vi "main_symulacyjny.vi"() -> ()   [LabVIEW 2020]
uses:
  Kontrolki/Parametry_cosinusow.ctl
  Kontrolki/Parametry_cosinusa.ctl
  Kontrolki/Rodzaj_wzmacniacza.ctl
  Kontrolki/Rodzaj_modulacji.ctl
  Kontrolki/Dane.ctl
  Kontrolki/Pasmo_przenoszenia.ctl
  <vilib>/measure/maspectr.llb/FFT Spectrum (Mag-Phase) for 1 Chan.vi
  <vilib>/measure/NI_MAPro.lvlib
panel:
  out "Widmo_sygnalu_zdemodulowanego":cluster{"f0":dbl, "df":dbl, "magnitude":dbl[]}(graph)
  out "Moc_szczytowa":dbl
  out "Sprawnosc":dbl
  out "Moc_srednia":dbl
  out "Energia_sygnalu_zmodulowanego":waveform(dbl)(graph) caption="Waveform Chart 2"
  out "Moc_sygnalu_zmodulowanego":waveform(dbl)(graph) caption="Waveform Chart 2"
  out "Widmo_sygnalu_zmodulowanego":cluster{"f0":dbl, "df":dbl, "magnitude":dbl[]}(graph)
  out "Sygnal_zmodulowany":waveform(dbl)(graph) caption="Waveform Chart 2"
  out "Widmo_sygnalu_modulujacego":cluster{"f0":dbl, "df":dbl, "magnitude":dbl[]}(graph)
  out "Sygnal_modulujacy_i_zdemodulowany":waveform(dbl)[](graph) caption="Waveform Chart 2"
  in  "Rodzaj_modulacji":T1
  in  "Parametry_sygnalu_nosnego":T2={"Amplituda [V]"=1.0, "Czestotliwosc [Hz] "=2.0, "Faza [rad]"=0.0}
  in  "Rodzaj_wzmacniacza":T3
  in  "Wzmocnienie":dbl=1.0
  in  "Milisekund_na_dane":u32=20
  in  "Parametry_sygnalu_modulujacego":T4 {"Czestotliwosc [Hz]" min=0.3 step=0.1}
  in  "stop":bool
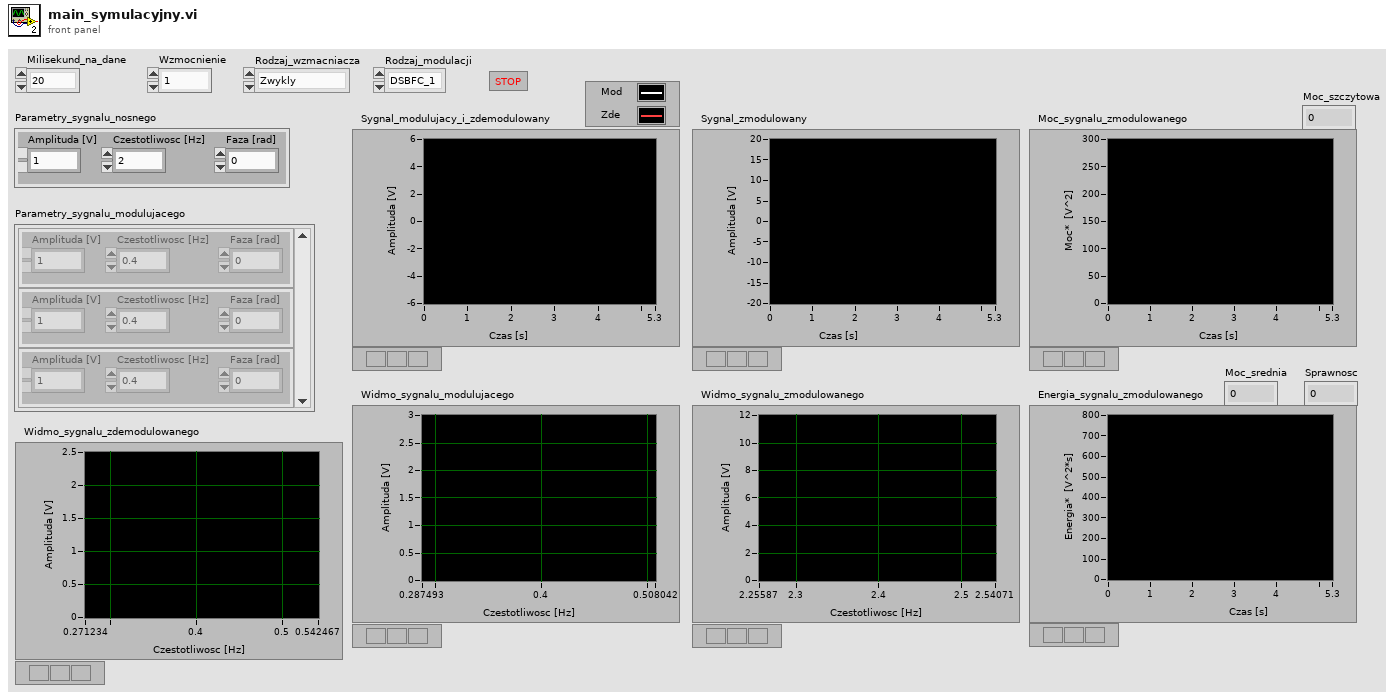
[diagram p1: front panel]
types:
  T1 = typedef "Rodzaj_modulacji.ctl" = enum16{"DSBFC_1", "DSBFC_2", "DSBSC", "USSBSC", "LSSBSC"}
  T2 = typedef "Parametry_cosinusa.ctl" = cluster{"Amplituda [V]":dbl, "Czestotliwosc [Hz] ":dbl, "Faza [rad]":dbl}
  T3 = typedef "Rodzaj_wzmacniacza.ctl" = enum16{"Zwykly", "Calkujacy", "Rozniczkujacy"}
  T4 = typedef "Parametry_cosinusow.ctl" = T2[]
  T5 = typedef "Dane.ctl" = cluster{"Parametry_sygnalu_modulujacego":T4, "Parametry_sygnalu_modulujacego_przesunietego":T4, "Sygnal_modulujacy_wzmocniony":dbl[], "Milisekund_na_dane":u32, "Wzmocnienie":dbl, "Rodzaj_wzmacniacza":T3, "Parametry_sygnalu_nosnego":T2, "Wektor_czasu":dbl[], "Sygnal_zmodulowany":dbl[], "Moc_sygnalu":dbl[], "Energia_sygnalu":dbl[], "Moc_szczytowa":dbl, "Sprawnosc":dbl, "Wartosc_poprzednia":dbl, "Czas":dbl, "Rodzaj_modulacji":T1, "Wartosc_poprzednia 2":dbl, "Moc_srednia":dbl, "Sygnal_zdemodulowany":dbl[], "Pasmo_przenoszenia":T6, "Rzeczywisty_sygnal":dbl[], "Rzeczywisty_zmodulowany":dbl[]}
  T6 = typedef "Pasmo_przenoszenia.ctl" = cluster{"f_L":dbl, "f_H":dbl}
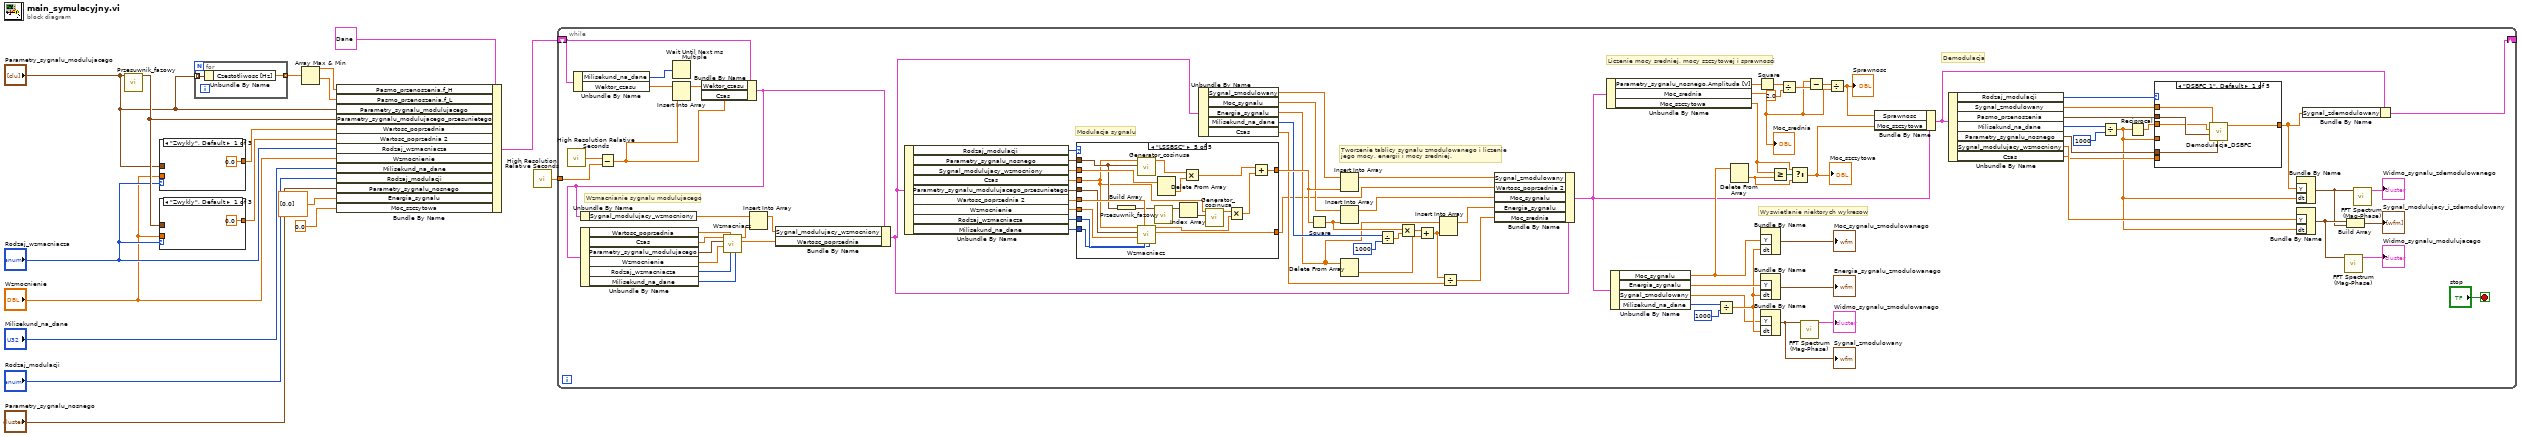
[diagram p0: block diagram]
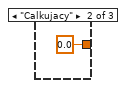
[diagram p2: hidden frame]
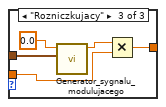
[diagram p3: hidden frame]
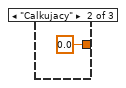
[diagram p4: hidden frame]
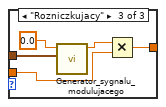
[diagram p5: hidden frame]
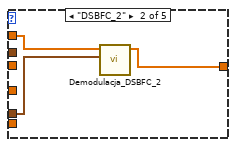
[diagram p6: hidden frame]
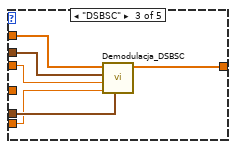
[diagram p7: hidden frame]
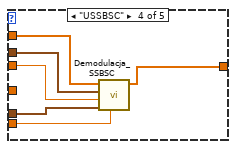
[diagram p8: hidden frame]
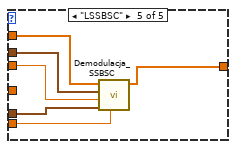
[diagram p9: hidden frame]
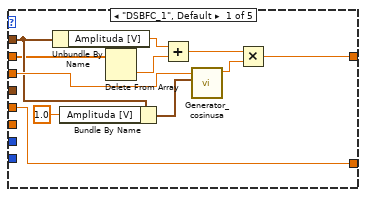
[diagram p10: hidden frame]
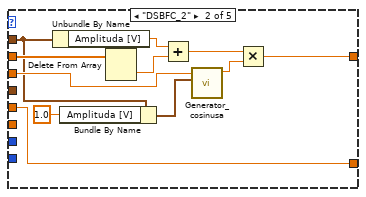
[diagram p11: hidden frame]
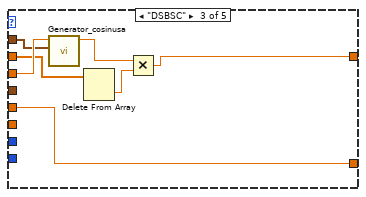
[diagram p12: hidden frame]
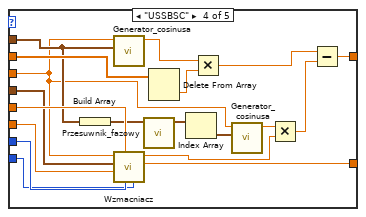
[diagram p13: hidden frame]
diagram:
  n1 = call "Przesuwnik_fazowy.vi"("Parametry_cosinusow"="Parametry_sygnalu_modulujacego") -> ("Parametry_cosinusow\nprzesuniete_w_fazie"=w9:T2[])  [unwired: 10 in]
  n2 = case shown="\"Zwykly\", Default" "Rodzaj_wzmacniacza" {
    tunnel: "Parametry_sygnalu_modulujacego" -> [_ _ w24]
    tunnel: [0.0 ("Sygnal_modulujacy") 0.0 ("Sygnal_modulujacy") w21] -> w11
    tunnel: "Wzmocnienie" -> [_ _ w20]
    frame "Zwykly", Default {
    }
    frame "Calkujacy" {
    }
    frame "Rozniczkujacy" {
      n3 = call "Generator_sygnalu_modulujacego.vi"("Parametry_cosinusow"=w24, "Czas"=0.0) -> ("Sygnal_modulujacy"=w22:dbl)  [unwired: 9 in]
      n4 = Multiply(x=w22, y=w20) -> (x*y=w21:dbl)
    }
  }
  n5 = case shown="\"Zwykly\", Default" "Rodzaj_wzmacniacza" {
    tunnel: w9 -> [_ _ w31]
    tunnel: [0.0 ("Sygnal_modulujacy") 0.0 ("Sygnal_modulujacy") w29] -> w10
    tunnel: "Wzmocnienie" -> [_ _ w27]
    frame "Zwykly", Default {
    }
    frame "Calkujacy" {
    }
    frame "Rozniczkujacy" {
      n6 = call "Generator_sygnalu_modulujacego.vi"("Parametry_cosinusow"=w31, "Czas"=0.0) -> ("Sygnal_modulujacy"=w28:dbl)  [unwired: 9 in]
      n7 = Multiply(x=w28, y=w27) -> (x*y=w29:dbl)
    }
  }
  n8 = for {
    tunnel: "Parametry_sygnalu_modulujacego" -> [w33] mode=indexing
    tunnel: [w32] -> w3 mode=indexing
    n9 = Unbundle By Name(w33) -> ("Czestotliwosc [Hz]"=w32:dbl)
  }
  n10 = Array Max & Min(array=w3) -> (max value=w1:dbl, min value=w2:dbl)  [unwired: 2 out]
  n11 = Bundle By Name(cluster=T5 {"Parametry_sygnalu_modulujacego"=[], "Parametry_sygnalu_modulujacego_przesunietego"=[], "Sygnal_modulujacy_wzmocniony"=[], "Milisekund_na_dane"=0, "Wzmocnienie"=0.0, "Rodzaj_wzmacniacza"=enum."Zwykly", "Parametry_sygnalu_nosnego"={"Amplituda [V]"=0.0, "Czestotliwosc [Hz] "=0.0, "Faza [rad]"=0.0}, "Wektor_czasu"=[], "Sygnal_zmodulowany"=[], "Moc_sygnalu"=[], "Energia_sygnalu"=[], "Moc_szczytowa"=0.0, "Sprawnosc"=0.0, "Wartosc_poprzednia"=0.0, "Czas"=0.0, "Rodzaj_modulacji"=enum."DSBFC_1", "Wartosc_poprzednia 2"=0.0, "Moc_srednia"=0.0, "Sygnal_zdemodulowany"=[], "Pasmo_przenoszenia"={"f_L"=0.0, "f_H"=0.0}, "Rzeczywisty_sygnal"=[], "Rzeczywisty_zmodulowany"=[]} ("Dane"), "Pasmo_przenoszenia.f_H"=w1, "Pasmo_przenoszenia.f_L"=w2, "Parametry_sygnalu_modulujacego"="Parametry_sygnalu_modulujacego", "Parametry_sygnalu_modulujacego_przesunietego"=w9, "Wartosc_poprzednia"=w11, "Wartosc_poprzednia 2"=w10, "Rodzaj_wzmacniacza"="Rodzaj_wzmacniacza", "Wzmocnienie"="Wzmocnienie", "Milisekund_na_dane"="Milisekund_na_dane", "Rodzaj_modulacji"="Rodzaj_modulacji", "Parametry_sygnalu_nosnego"="Parametry_sygnalu_nosnego", "Energia_sygnalu"=dbl[] [0.0], "Moc_szczytowa"=0.0) -> (w14:T5)
  n12 = call <vilib>:"High Resolution Relative Seconds.vi"() -> ("relative seconds"=w13:dbl)
  n13 = while {
    shift-right: [w37] -> _
    shift-left: w14 -> [w114]
    tunnel: w13 -> [w118]
    stop <- "stop" stop-if-true
    # "Wzmacnianie sygnalu modulujacego"
    # "Liczenie mocy sredniej, mocy szczytowej i sprawnosci"
    # "Wyswietlanie niektorych wykresow"
    # "Tworzenie tablicy sygnalu zmodulowanego i liczenie\njego mocy, energii i mocy sredniej."
    # "Demodulacja"
    # "Modulacja sygnalu"
    n14 = call <vilib>:"High Resolution Relative Seconds.vi"() -> ("relative seconds"=w119:dbl)
    n15 = Unbundle By Name(w114) -> ("Milisekund_na_dane"=w115:u32, "Wektor_czasu"=w117:dbl[])
    n16 = Subtract(x=w119, y=w118) -> (x-y=w113:dbl)
    n17 = Wait Until Next ms Multiple(millisecond multiple=w115) -> ()  [unwired: 1 out]
    n18 = Insert Into Array(array=w117, new element=w113) -> (w116:dbl[])  [unwired: 1 in]
    n19 = Bundle By Name(cluster=w114, "Wektor_czasu"=w116, "Czas"=w113) -> (w100:T5)
    n20 = Unbundle By Name(w100) -> ("Wartosc_poprzednia"=w112:dbl, "Czas"=w93:dbl, "Parametry_sygnalu_modulujacego"=w92:T4, "Wzmocnienie"=w109:dbl, "Rodzaj_wzmacniacza"=w110:T3, "Milisekund_na_dane"=w111:u32)
    n21 = Unbundle By Name(w100) -> ("Sygnal_modulujacy_wzmocniony"=w99:dbl[])
    n22 = call "Wzmacniacz.vi"("Milisekund_na_dane"=w111, "Rodzaj_wzmacniacza"=w110, "Wartosc_poprzednia"=w112, "Wzmocnienie"=w109, "Parametry_cosinusow"=w92, "Czas"=w93) -> ("Wartosc_poprzednia"=w91:dbl, "Sygnal_wzmocniony"=w90:dbl)  [unwired: 4 in]
    n23 = Insert Into Array(array=w99, new element=w90) -> (w98:dbl[])  [unwired: 1 in]
    n24 = Bundle By Name(cluster=w100, "Sygnal_modulujacy_wzmocniony"=w98, "Wartosc_poprzednia"=w91) -> (w97:T5)
    n25 = Unbundle By Name(w97) -> ("Rodzaj_modulacji"=w105:T1, "Parametry_sygnalu_nosnego"=w108:T2, "Sygnal_modulujacy_wzmocniony"=w96:dbl[], "Czas"=w107:dbl, "Parametry_sygnalu_modulujacego_przesunietego"=w106:T4, "Wartosc_poprzednia 2"=w104:dbl, "Wzmocnienie"=w103:dbl, "Rodzaj_wzmacniacza"=w102:T3, "Milisekund_na_dane"=w101:u32)
    n26 = case shown="\"LSSBSC\"" w105 {
      tunnel: w108 -> [w153 w160 w173 w183 w202]
      tunnel: w96 -> [w148 w163 w170 w191 w210]
      tunnel: w107 -> [w154 w161 w174 w179 w198]
      tunnel: [w146 w164 w169 w190 w209] -> w87
      tunnel: w106 -> [_ _ _ w187 w206]
      tunnel: w104 -> [w150 w157 w168 w188 w207]
      tunnel: w103 -> [_ _ _ w186 w205]
      tunnel: w102 -> [_ _ _ w185 w204]
      tunnel: w101 -> [_ _ _ w184 w203]
      tunnel: [w150 w157 w168 w178 w197] -> w62
      frame "DSBFC_1", Default {
        n27 = Unbundle By Name(w153) -> ("Amplituda [V]"=w156:dbl)
        n28 = Bundle By Name(cluster=w153, "Amplituda [V]"=1.0) -> (w151:T2)
        n29 = Delete From Array(array=w148) -> (deleted portion=w149:dbl)  [unwired: 2 in, 1 out]
        n30 = Add(x=w156, y=w149) -> (x+y=w147:dbl)
        n31 = call "Generator_cosinusa.vi"("Parametry_cosinusa"=w151, "Czas"=w154) -> ("A cos(2pift + phi)"=w155:dbl)  [unwired: 9 in]
        n32 = Multiply(x=w147, y=w155) -> (x*y=w146:dbl)
      }
      frame "DSBFC_2" {
        n33 = Unbundle By Name(w160) -> ("Amplituda [V]"=w167:dbl)
        n34 = Bundle By Name(cluster=w160, "Amplituda [V]"=1.0) -> (w158:T2)
        n35 = Delete From Array(array=w163) -> (deleted portion=w162:dbl)  [unwired: 2 in, 1 out]
        n36 = Add(x=w167, y=w162) -> (x+y=w166:dbl)
        n37 = call "Generator_cosinusa.vi"("Parametry_cosinusa"=w158, "Czas"=w161) -> ("A cos(2pift + phi)"=w165:dbl)  [unwired: 9 in]
        n38 = Multiply(x=w166, y=w165) -> (x*y=w164:dbl)
      }
      frame "DSBSC" {
        n39 = call "Generator_cosinusa.vi"("Parametry_cosinusa"=w173, "Czas"=w174) -> ("A cos(2pift + phi)"=w172:dbl)  [unwired: 9 in]
        n40 = Delete From Array(array=w170) -> (deleted portion=w171:dbl)  [unwired: 2 in, 1 out]
        n41 = Multiply(x=w172, y=w171) -> (x*y=w169:dbl)
      }
      frame "USSBSC" {
        n42 = Build Array(w183) -> (w182:T2[])
        n43 = call "Generator_cosinusa.vi"("Parametry_cosinusa"=w183, "Czas"=w179) -> ("A cos(2pift + phi)"=w193:dbl)  [unwired: 9 in]
        n44 = call "Wzmacniacz.vi"("Milisekund_na_dane"=w184, "Rodzaj_wzmacniacza"=w185, "Wartosc_poprzednia"=w188, "Wzmocnienie"=w186, "Parametry_cosinusow"=w187, "Czas"=w179) -> ("Wartosc_poprzednia"=w178:dbl, "Sygnal_wzmocniony"=w176:dbl)  [unwired: 4 in]
        n45 = call "Przesuwnik_fazowy.vi"("Parametry_cosinusow"=w182) -> ("Parametry_cosinusow\nprzesuniete_w_fazie"=w181:T2[])  [unwired: 10 in]
        n46 = Delete From Array(array=w191) -> (deleted portion=w192:dbl)  [unwired: 2 in, 1 out]
        n47 = Index Array(array=w181) -> (element=w180:T2)  [unwired: 1 in]
        n48 = Multiply(x=w193, y=w192) -> (x*y=w189:dbl)
        n49 = call "Generator_cosinusa.vi"("Parametry_cosinusa"=w180, "Czas"=w179) -> ("A cos(2pift + phi)"=w177:dbl)  [unwired: 9 in]
        n50 = Multiply(x=w177, y=w176) -> (x*y=w175:dbl)
        n51 = Subtract(x=w189, y=w175) -> (x-y=w190:dbl)
      }
      frame "LSSBSC" {
        n52 = Build Array(w202) -> (w201:T2[])
        n53 = call "Generator_cosinusa.vi"("Parametry_cosinusa"=w202, "Czas"=w198) -> ("A cos(2pift + phi)"=w212:dbl)  [unwired: 9 in]
        n54 = call "Wzmacniacz.vi"("Milisekund_na_dane"=w203, "Rodzaj_wzmacniacza"=w204, "Wartosc_poprzednia"=w207, "Wzmocnienie"=w205, "Parametry_cosinusow"=w206, "Czas"=w198) -> ("Wartosc_poprzednia"=w197:dbl, "Sygnal_wzmocniony"=w195:dbl)  [unwired: 4 in]
        n55 = call "Przesuwnik_fazowy.vi"("Parametry_cosinusow"=w201) -> ("Parametry_cosinusow\nprzesuniete_w_fazie"=w200:T2[])  [unwired: 10 in]
        n56 = Delete From Array(array=w210) -> (deleted portion=w211:dbl)  [unwired: 2 in, 1 out]
        n57 = Index Array(array=w200) -> (element=w199:T2)  [unwired: 1 in]
        n58 = Multiply(x=w212, y=w211) -> (x*y=w208:dbl)
        n59 = call "Generator_cosinusa.vi"("Parametry_cosinusa"=w199, "Czas"=w198) -> ("A cos(2pift + phi)"=w196:dbl)  [unwired: 9 in]
        n60 = Multiply(x=w196, y=w195) -> (x*y=w194:dbl)
        n61 = Add(x=w208, y=w194) -> (x+y=w209:dbl)
      }
    }
    n62 = Unbundle By Name(w97) -> ("Sygnal_zmodulowany"=w94:dbl[], "Moc_sygnalu"=w86:dbl[], "Energia_sygnalu"=w76:dbl[], "Milisekund_na_dane"=w80:u32, "Czas"=w73:dbl)
    n63 = Square(x=w87) -> (x^2=w82:dbl)
    n64 = Insert Into Array(array=w94, new element=w87) -> (w95:dbl[])  [unwired: 1 in]
    n65 = Insert Into Array(array=w86, new element=w82) -> (w85:dbl[])  [unwired: 1 in]
    n66 = Delete From Array(array=w76) -> (deleted portion=w77:dbl)  [unwired: 2 in, 1 out]
    n67 = Divide(x=w80, y=1000) -> (x/y=w79:dbl)
    n68 = Multiply(x=w82, y=w79) -> (x*y=w78:dbl)
    n69 = Add(x=w78, y=w77) -> (x+y=w72:dbl)
    n70 = Insert Into Array(array=w76, new element=w72) -> (w75:dbl[])  [unwired: 1 in]
    n71 = Divide(x=w72, y=w73) -> (x/y=w71:dbl)
    n72 = Bundle By Name(cluster=w97, "Sygnal_zmodulowany"=w95, "Wartosc_poprzednia 2"=w62, "Moc_sygnalu"=w85, "Energia_sygnalu"=w75, "Moc_srednia"=w71) -> (w36:T5)
    n73 = Unbundle By Name(w36) -> ("Parametry_sygnalu_nosnego.Amplituda [V]"=w57:dbl, "Moc_srednia"=w52:dbl, "Moc_szczytowa"=w68:dbl)
    "Moc_srednia" <- w52
    n74 = Unbundle By Name(w36) -> ("Moc_sygnalu"=w70:dbl[], "Energia_sygnalu"=w60:dbl[], "Sygnal_zmodulowany"=w38:dbl[], "Milisekund_na_dane"=w61:u32)
    n75 = Divide(x=w61, y=1000) -> (x/y=w59:dbl)
    n76 = Delete From Array(array=w70) -> (deleted portion=w58:dbl)  [unwired: 2 in, 1 out]
    n77 = Square(x=w57) -> (x^2=w56:dbl)
    n78 = Bundle By Name("Y"=w70, "dt"=w59) -> (→"Moc_sygnalu_zmodulowanego":waveform(dbl))  [unwired: 1 in]
    n79 = Bundle By Name("Y"=w60, "dt"=w59) -> (→"Energia_sygnalu_zmodulowanego":waveform(dbl))  [unwired: 1 in]
    n80 = Bundle By Name("Y"=w38, "dt"=w59) -> (w34:waveform(dbl))  [unwired: 1 in]
    "Sygnal_zmodulowany" <- w34
    n81 = Greater Or Equal?(x=w68, y=w58) -> (x >= y?=w69:bool)
    n82 = Divide(x=w56, y=2.0) -> (x/y=w54:dbl)
    n83 = Select(t=w68, s=w69, f=w58) -> (s? t:f=w67:dbl)
    "Moc_szczytowa" <- w67
    n84 = call-poly <vilib>:"FFT Spectrum (Mag-Phase).vi"("time signal"=w34) -> ("magnitude"=→"Widmo_sygnalu_zmodulowanego":cluster{"f0":dbl, "df":dbl, "magnitude":dbl[]})  [unwired: 6 in, 4 out]
    n85 = Subtract(x=w52, y=w54) -> (x-y=w53:dbl)
    n86 = Divide(x=w53, y=w52) -> (x/y=w49:dbl)
    "Sprawnosc" <- w49
    n87 = Bundle By Name(cluster=w36, "Sprawnosc"=w49, "Moc_szczytowa"=w67) -> (w63:T5)
    n88 = Unbundle By Name(w63) -> ("Rodzaj_modulacji"=w43:T1, "Sygnal_zmodulowany"=w47:dbl[], "Pasmo_przenoszenia"=w46:T6, "Milisekund_na_dane"=w65:u32, "Parametry_sygnalu_nosnego"=w44:T2, "Sygnal_modulujacy_wzmocniony"=w45:dbl[], "Czas"=w41:dbl)
    n89 = Divide(x=w65, y=u32 1000) -> (x/y=w35:dbl)
    n90 = Reciprocal(x=w35) -> (1/x=w42:dbl)
    n91 = case shown="\"DSBFC_1\", Default" w43 {
      tunnel: w47 -> [w124 w126 w129 w139 w145]
      tunnel: w46 -> [w123 _ w131 w138 w144]
      tunnel: w44 -> [w122 w127 w133 w135 w141]
      tunnel: [w121 w125 w128 w137 w143] -> w40
      tunnel: w42 -> [w120 _ w130 w136 w142]
      tunnel: w35 -> [_ _ _ _ _]
      tunnel: w41 -> [_ _ w132 w134 w140]
      frame "DSBFC_1", Default {
        n92 = call "Demodulacja_DSBFC.vi"("Parametry_sygnalu_nosnego"=w122, "Pasmo_przenoszenia"=w123, "Czestotliwosc_probkowania"=w120, "Sygnal_zmodulowany"=w124) -> ("Sygnal_zdemodulowany"=w121:dbl[])  [unwired: 7 in]
      }
      frame "DSBFC_2" {
        n93 = call "Demodulacja_DSBFC_2.vi"("Parametry_sygnalu_nosnego"=w127, "Sygnal_zmodulowany"=w126) -> ("Sygnal_zdemodulowany"=w125:dbl[])  [unwired: 9 in]
      }
      frame "DSBSC" {
        n94 = call "Demodulacja_DSBSC.vi"("Sygnal_zmodulowany"=w129, "Pasmo_przenoszenia"=w131, "Czestotliwosc_probkowania"=w130, "Czas"=w132, "Parametry_sygnalu_nosnego"=w133) -> ("Sygnal_zdemodulowany"=w128:dbl[])  [unwired: 5 in]
      }
      frame "USSBSC" {
        n95 = call "Demodulacja_SSBSC.vi"("Czas"=w134, "Parametry_sygnalu_nosnego"=w135, "Czestotliwosc_probkowania"=w136, "Pasmo_przenoszenia"=w138, "Sygnal_zmodulowany"=w139) -> ("Sygnal_zdemodulowany"=w137:dbl[])  [unwired: 6 in]
      }
      frame "LSSBSC" {
        n96 = call "Demodulacja_SSBSC.vi"("Czas"=w140, "Parametry_sygnalu_nosnego"=w141, "Czestotliwosc_probkowania"=w142, "Pasmo_przenoszenia"=w144, "Sygnal_zmodulowany"=w145) -> ("Sygnal_zdemodulowany"=w143:dbl[])  [unwired: 6 in]
      }
    }
    n97 = Bundle By Name("Y"=w40, "dt"=w35) -> (w39:waveform(dbl))  [unwired: 1 in]
    n98 = Bundle By Name("Y"=w45, "dt"=w35) -> (w51:waveform(dbl))  [unwired: 1 in]
    n99 = Bundle By Name(cluster=w63, "Sygnal_zdemodulowany"=w40) -> (w37:T5)
    n100 = call-poly <vilib>:"FFT Spectrum (Mag-Phase).vi"("time signal"=w51) -> ("magnitude"=→"Widmo_sygnalu_modulujacego":cluster{"f0":dbl, "df":dbl, "magnitude":dbl[]})  [unwired: 6 in, 4 out]
    n101 = Build Array(w51, w39) -> (→"Sygnal_modulujacy_i_zdemodulowany":waveform(dbl)[])
    n102 = call-poly <vilib>:"FFT Spectrum (Mag-Phase).vi"("time signal"=w39) -> ("magnitude"=→"Widmo_sygnalu_zdemodulowanego":cluster{"f0":dbl, "df":dbl, "magnitude":dbl[]})  [unwired: 6 in, 4 out]
  }
